vi "USB RAW - Control.vi"() -> ()   [LabVIEW 2023]
doc: "This example shows how to perform control pipe transfers to and from a USB RAW device as results of user events. \n\n<b>Note:</b> This example works only with USB RAW devices.\n\nBefore you run this VI, install a USB RAW device and configure NI Measurement & Automation Explorer (MAX) to recognize the USB device. You can perform control pipe transfers to and from the USB RAW device only after you install and configure the USB RAW device and open a session to the device.\n\nThis VI reads the values of the data payload from the <b>RequestType</b>, <b>Request</b>, <b>Value</b>, <b>Index</b>, and <b>Length</b> fields. The values you enter in these fields depend largely on the USB RAW device. However, there are a few standard calls that you can make. For example, you can enter the following values to get the status of a particular device:\n\n<b>Request Type</b>: 0x80 (Device to Host, Standard Type, Device Recipient)\n<b>Request</b>: 0x00 (GET_STATUS)\n<b>Value</b>: 0x00 \n<b>Index</b>: 0x00\n<b>Length</b>: 0x02\n\n<b>Note:</b> The previous fields accept values in hexadecimal format by default. Right-click a field and select <b>Display Format</b> from the shortcut menu to change the format of the values that field accepts. \n\nThe last two bits of the value this VI returns indicate whether the device is set to remotely wake up (bit 1) and whether the device is self-powered (bit 0). \n\nTo perform control transfers with another device, close the session to the current device, select another device from the <b>VISA Resource</b> control and open a session to the new device. \n\nWhen the control pipe transfer is complete, click the <b>Stop</b> button to stop the VI."
panel:
  in  "Not USB":string="The specified VISA resource is not a USB device."
  out "Length returned":i32
  in  "Index":u16 format="%.0x"
  in  "Value":u16 format="%.0x"
  in  "Request":i16 format="%.0x"
  in  "Request Type":i16 format="%.0x"
  in  "Length":u16=5
  out "Control In Buffer":u8[](array[numeric])
  in  "Control Out Buffer":u8[](array[numeric])
  in  "Stop":bool
  in  "VISA Resource":refnum<visa-resource-name>
  in  "Control In":bool
  in  "Control Out":bool
  # "Overview: Demonstrates the use of the VISA USB functions to communicate with a USB RAW device.\nRequirements: NI-VISA Driver, USB RAW device\nInstructions:\n1. Ensure the USB RAW device specified by the VISA Resource control is properly configured in Measurement & Automation Explorer.\n2. Run the VI.\n3. Ensure the Request Type, Request, Value, and Index values are valid.\n4. Click the Control Out and Control In buttons to write to/read from your USB RAW device.\n5. Click Stop to stop the VI."
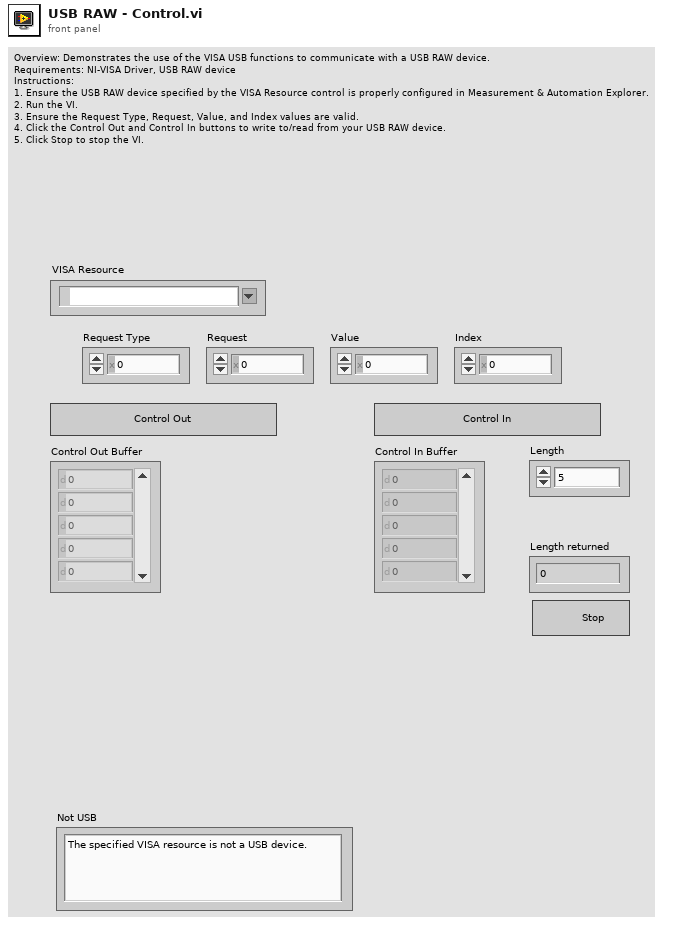
[diagram p1: front panel]
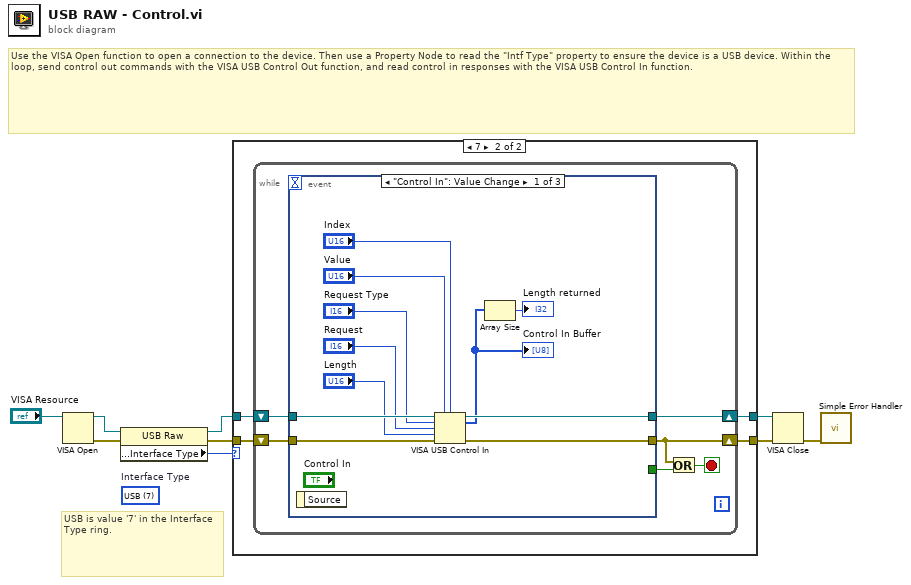
[diagram p0: block diagram]
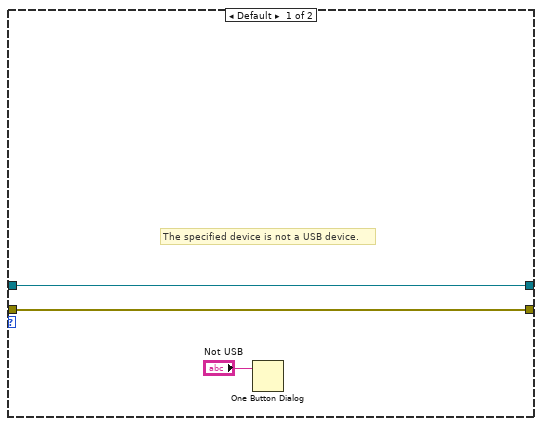
[diagram p2: hidden frame]
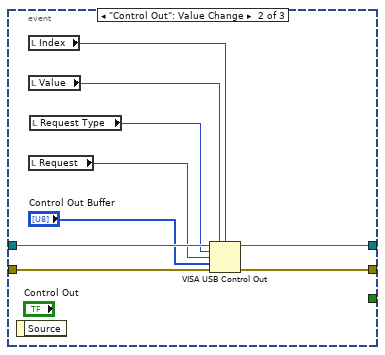
[diagram p3: hidden frame]
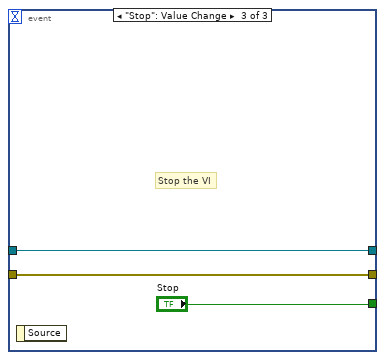
[diagram p4: hidden frame]
diagram:
  (unwired) u16 7 items=["GPIB"=1, "VXI"=2, "GPIB-VXI"=3, "Serial"=4, "PXI"=5, "TCPIP"=6, "USB"=7, "FireWire"=9]  # Interface Type
  # "Use the VISA Open function to open a connection to the device. Then use a Property Node to read the \"Intf Type\" property to ensure the device is a USB device. Within the loop, send control out commands with the VISA USB Control Out function, and read control in responses with the VISA USB Control In function."
  # "USB is value '7' in the Interface Type ring."
  n1 = VISA Open(VISA resource name="VISA Resource") -> (VISA resource name=w6:refnum<visa-resource-name>, error out=w5:errorcluster)  [unwired: 1 in, 3 out]
  n2 = property class="USB Raw"(reference=w6, error in=w5) -> (reference out=w3:refnum<visa-resource-name>, error out=w4:errorcluster, "Interface Information:Interface Type"=w1:u16)
  n3 = case shown="7" w1 {
    tunnel: [w11 w16] -> w9
    tunnel: [w12 w15] -> w7
    tunnel: w4 -> [w11 w14]
    tunnel: w3 -> [w12 w13]
    frame Default {
      # "The specified device is not a USB device."
      n4 = One Button Dialog(message="Not USB") -> ()  [unwired: 1 in, 1 out]
    }
    frame 7 {
      n5 = while {
        shift-right: [w17] -> w16
        shift-left: w14 -> [w18]
        shift-right: [w20] -> w15
        shift-left: w13 -> [w19]
        stop <- w21 stop-if-true
        n6 = event shown="[0] \"Control In\": Value Change" {
          selector: _ -> [_ _ _]
          dyn-events: _ -> [_ _ _]
          timeout: _ -> [_ _ _]
          tunnel: [_ _ "Stop"] -> w22
          tunnel: [w33 w40 w44] -> w17
          tunnel: w18 -> [w30 w41 w44]
          tunnel: [w32 w39 w43] -> w20
          tunnel: w19 -> [w31 w42 w43]
          event "Control In": Value Change {
            n7 = event-data() -> ()  [unwired: 2 out]
            n8 = VISA USB Control In(0:w31, 1:"Value", 2:"Index", 5:"Request Type", 7:"Request", 9:"Length", 11:w30) -> (4:w32:refnum<visa-resource-name>, 6:w23:u8[], 15:w33:errorcluster)
            "Control In Buffer" <- w23
            n9 = Array Size(array=w23) -> (size(s)=→"Length returned":i32)
          }
          event "Control Out": Value Change {
            n10 = event-data() -> ()  [unwired: 2 out]
            n11 = local read "Index"() -> (w38:u16)
            n12 = local read "Value"() -> (w37:u16)
            n13 = local read "Request"() -> (w35:i16)
            n14 = local read "Request Type"() -> (w36:i16)
            n15 = VISA USB Control Out(0:w42, 1:w37, 2:w38, 5:w36, 7:w35, 9:"Control Out Buffer", 11:w41) -> (4:w39:refnum<visa-resource-name>, 15:w40:errorcluster)
          }
          event "Stop": Value Change {
            # "Stop the VI"
            n16 = event-data() -> ()  [unwired: 2 out]
          }
        }
        n17 = Or(x=w17, y=w22) -> (x .or. y?=w21:bool)
      }
    }
  }
  n18 = VISA Close(VISA resource name=w7, error in (no error)=w9) -> (error out=w8:errorcluster)
  n19 = call <vilib>:"Simple Error Handler.vi"("error in (no error)"=w8) -> ()  [unwired: 1 in, 8 out]
